vi "Cleanup.vi"(8 "error in (no error)":errorcluster, 11 "CDependencyInspection in":refnum<class "CDependencyInspection.lvclass">) -> (0 "error out":errorcluster, 3 "CDependencyInspection out":refnum<class "CDependencyInspection.lvclass">)   [LabVIEW 2020, in "DependencyInspection.lvlib" / "CDependencyInspection.lvclass"]
uses:
  CDependencyInspection.lvclass
  CDependencyList/CDependencyList.lvclass
  CRuleList/CRuleList.lvclass
  CReporter/CReporter.lvclass
  obj/Addons/ErrorManager.lvlibp/ErrorManager/ErrorManager.lvclass
  CDebugInfo/CDebugInfo.lvclass
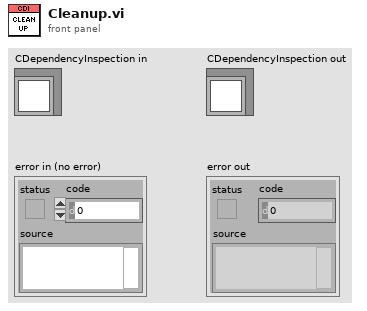
[diagram p1: front panel]
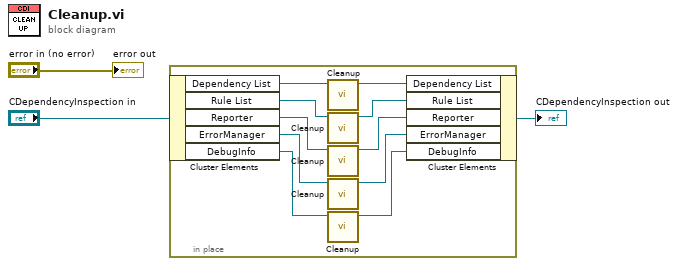
[diagram p0: block diagram]
diagram:
  n1 = in-place {
    n2 = in-place-cluster #1("CDependencyInspection in") -> ("Dependency List"=w13:refnum<class "CDependencyList.lvclass">, "Rule List"=w11:refnum<class "CRuleList.lvclass">, "Reporter"=w9:refnum<class "CReporter.lvclass">, "ErrorManager"=w8:refnum<class "ErrorManager.lvclass">, "DebugInfo"=w7:refnum<class "CDebugInfo.lvclass">)
    n3 = call-dynamic "Cleanup.vi"("CDependencyList in"=w13) -> ("CDependencyList out"=w12:refnum<class "CDependencyList.lvclass">)  [unwired: 9 in, 1 out]
    n4 = call-dynamic "Cleanup.vi"("CRuleList in"=w11) -> ("CRuleList out"=w10:refnum<class "CRuleList.lvclass">)  [unwired: 9 in, 1 out]
    n5 = call-dynamic "Cleanup.vi"("CReporter in"=w9) -> ("CReporter out"=w6:refnum<class "CReporter.lvclass">)  [unwired: 9 in, 1 out]
    n6 = call-dynamic "Cleanup.vi"("ErrorManager in"=w8) -> ("ErrorManager out"=w5:refnum<class "ErrorManager.lvclass">)  [unwired: 9 in, 1 out]
    n7 = call-dynamic "Cleanup.vi"("CDebugInfo in"=w7) -> ("CDebugInfo out"=w4:refnum<class "CDebugInfo.lvclass">)  [unwired: 9 in, 1 out]
    n8 = in-place-cluster #1("Dependency List"=w12, "Rule List"=w10, "Reporter"=w6, "ErrorManager"=w5, "DebugInfo"=w4) -> (→"CDependencyInspection out":refnum<class "CDependencyInspection.lvclass">)
  }
  "error out" <- "error in (no error)"
